vi "Support Get Thermals.vi"(6 "Water Outlet Valve":i32, 8 "error in":errorcluster, 10 "Input Data":T16, 11 "All Data":T1 {"PLC Data"."PLC Data - LDO"."Timing"."Absolute Time" format="%<%H:%M:%S%3u>t"; "PLC Data"."PLC Data - LDO"."Timing"."Display Time" format="%#.20f"; "PLC Data"."PLC Data - LDO"."Timing"."Test Time Ref" format="%#.20f"; "PLC Data"."PLC Data - LDO"."Timing"."Precondition Time Ref" format="%#.20f"; "PLC Data"."PLC Data - LDO"."Timing"."First Call Time Ref" format="%#.20f"; "PLC Data"."PLC Data - FVIR"."Timing"."Absolute Time" format="%<%H:%M:%S%3u>t"; "PLC Data"."PLC Data - FVIR"."Timing"."Display Time" format="%#.20f"; "PLC Data"."PLC Data - FVIR"."Timing"."Test Time Ref" format="%#.20f"; "PLC Data"."PLC Data - FVIR"."Timing"."Precondition Time Ref" format="%#.20f"; "PLC Data"."PLC Data - FVIR"."Timing"."First Call Time Ref" format="%#.20f"}) -> (0 "error out":errorcluster, 3 "All Data Out":T1 {"PLC Data"."PLC Data - LDO"."Timing"."Absolute Time" format="%<%H:%M:%S%3u>t"; "PLC Data"."PLC Data - LDO"."Timing"."Display Time" format="%#.20f"; "PLC Data"."PLC Data - LDO"."Timing"."Test Time Ref" format="%#.20f"; "PLC Data"."PLC Data - LDO"."Timing"."Precondition Time Ref" format="%#.20f"; "PLC Data"."PLC Data - LDO"."Timing"."First Call Time Ref" format="%#.20f"; "PLC Data"."PLC Data - FVIR"."Timing"."Absolute Time" format="%<%H:%M:%S%3u>t"; "PLC Data"."PLC Data - FVIR"."Timing"."Display Time" format="%#.20f"; "PLC Data"."PLC Data - FVIR"."Timing"."Test Time Ref" format="%#.20f"; "PLC Data"."PLC Data - FVIR"."Timing"."Precondition Time Ref" format="%#.20f"; "PLC Data"."PLC Data - FVIR"."Timing"."First Call Time Ref" format="%#.20f"})   [LabVIEW 2023]
uses:
  Modbus/Modbus All Data.ctl
  Modbus/Modbus PLC Data All.ctl
  Modbus/Modbus FVIR Control.ctl
  Modbus/Modbus Timing.ctl
  <vilib>/Utility/miscctls.llb/LVDateTimeRec.ctl
  Modbus/Modbus LDO Control.ctl
  WritingDataFile/Data to Save.ctl
  Terminate Conditions Cluster.ctl
  Drivers/Inficon Transmitter/Type Definitions/Inficon Data.ctl
  Modbus/Modbus Gas Meter Data.ctl
  Drivers/Alicat LabVIEW Drivers 2v1/Sub-VIs/Data Cluster.ctl
  Drivers/Alicat LabVIEW Drivers 2v1/Sub-VIs/Units of Measure.ctl
  Gas_Rate/HEWH ANSI Rate.ctl
  Drivers/Resideo Gas Valve/Type Definitions/Vesta Info.ctl
  Agilent Data.ctl
  Thermal Calculation Cluster.ctl
panel:
  # "Totalizer Timer"
  # "Totalizer Timer"
  # "Natural Gas"
  # "Propane"
  # "Totalizer Timer"
  # "Totalizer Timer"
  # "Natural Gas"
  # "Propane"
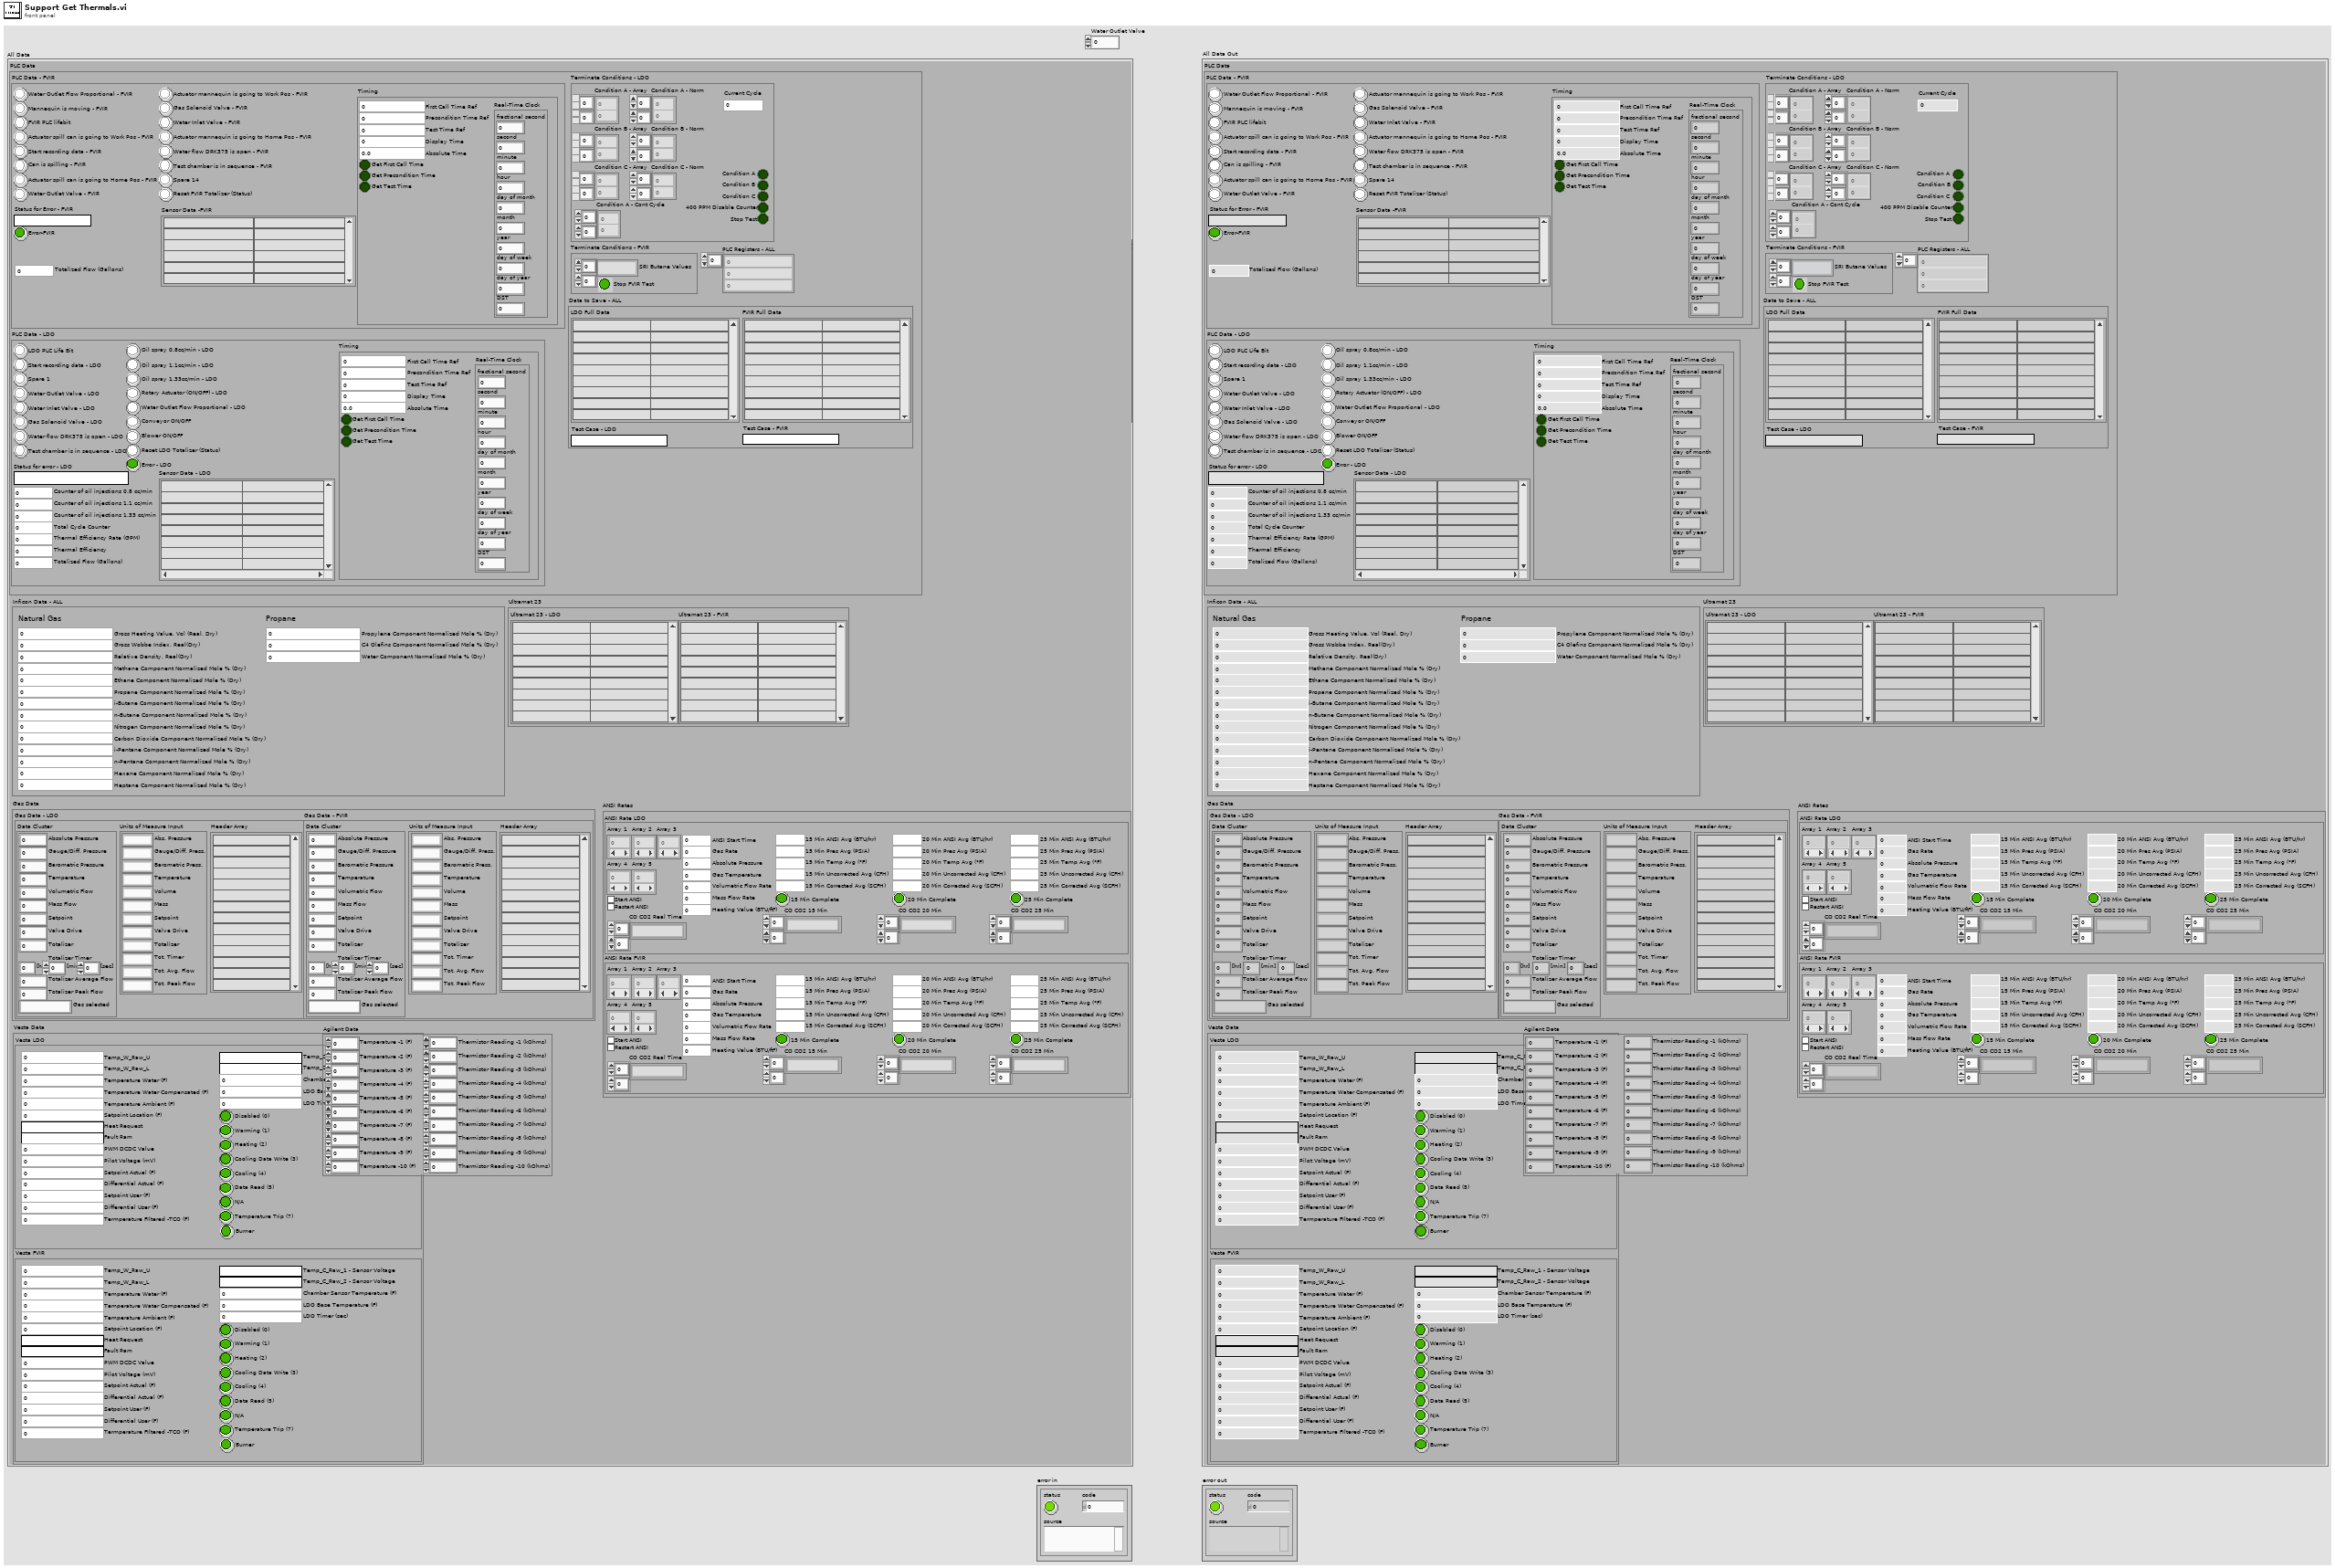
[diagram p1: front panel]
types:
  T1 = typedef "Modbus All Data.ctl" = cluster{"PLC Data":T2, "Inficon Data - ALL":T9, "Gas Data":cluster{"Gas Data - LDO":T10, "Gas Data - FVIR":T10}, "Ultramat 23":cluster{"Ultramat 23 - LDO":string[][], "Ultramat 23 - FVIR":string[][]}, "ANSI Rates":cluster{"ANSI Rate LDO":T13, "ANSI Rate FVIR":T13}, "Vesta Data":cluster{"Vesta LDO":T14, "Vesta FVIR":T14}, "Agilent Data":T15}
  T2 = typedef "Modbus PLC Data All.ctl" = cluster{"PLC Data - FVIR":T3, "PLC Data - LDO":T6, "PLC Registers - ALL":i16[], "Data to Save - ALL":T7, "Terminate Conditions - LDO":T8, "Terminate Conditions - FVIR":cluster{"SRI Butane Values":string[][], "Stop FVIR Test":bool}}
  T3 = typedef "Modbus FVIR Control.ctl" = cluster{"Reset FVIR Totalizer (Status)":bool, "Spare 14":bool, "Actuator mannequin is going to Work Pos - FVIR":bool, "Actuator mannequin is going to Home Pos - FVIR":bool, "Test chamber is in sequence - FVIR ":bool, "Water flow DRK375 is open - FVIR":bool, "Gas Solenoid Valve - FVIR":bool, "Water Inlet Valve - FVIR":bool, "Water Outlet Flow Proportional - FVIR":bool, "Start recording data - FVIR":bool, "Actuator spill can is going to Work Pos - FVIR":bool, "Actuator spill can is going to Home Pos - FVIR":bool, "Water Outlet Valve - FVIR":bool, "Can is spilling - FVIR":bool, "Mannequin is moving - FVIR":bool, "FVIR PLC lifebit":bool, "Status for Error - FVIR":string, "Error-FVIR":bool, "Sensor Data -FVIR":string[][], "Totalized Flow (Gallons)":dbl, "Timing":T4}
  T4 = typedef "Modbus Timing.ctl" = cluster{"First Call Time Ref":dbl, "Precondition Time Ref":dbl, "Test Time Ref":dbl, "Get First Call Time":bool, "Get Precondition Time":bool, "Get Test Time":bool, "Display Time":dbl, "Real-Time Clock":T5, "Absolute Time":dbl}
  T5 = typedef "LVDateTimeRec.ctl" = cluster{"fractional second":dbl, "second":i32, "minute":i32, "hour":i32, "day of month":i32, "month":i32, "year":i32, "day of week":i32, "day of year":i32, "DST":i32}
  T6 = typedef "Modbus LDO Control.ctl" = cluster{"LDO PLC Life Bit":bool, "Start recording data - LDO":bool, "Spare 1":bool, "Water Outlet Valve - LDO":bool, "Water Inlet Valve - LDO":bool, "Gas Solenoid Valve - LDO":bool, "Water flow DRK375 is open - LDO":bool, "Test chamber is in sequence - LDO":bool, "Oil spray 0.8cc/min - LDO":bool, "Oil spray 1.1cc/min - LDO":bool, "Oil spray 1.33cc/min - LDO":bool, "Rotary Actuator (ON/OFF) - LDO":bool, "Water Outlet Flow Proportional - LDO":bool, "Conveyor ON/OFF":bool, "Blower ON/OFF":bool, "Reset LDO Totalizer (Status)":bool, "Status for error - LDO":string, "Error - LDO":bool, "Sensor Data - LDO":string[][], "Thermal Efficiency Rate (GPM)":dbl, "Thermal Efficiency":dbl, "Totalized Flow (Gallons)":dbl, "Counter of oil injections 1.33 cc/min":u16, "Total Cycle Counter":u16, "Counter of oil injections 1.1 cc/min":u16, "Counter of oil injections 0.8 cc/min":u16, "Timing":T4}
  T7 = typedef "Data to Save.ctl" = cluster{"LDO Full Data":string[][], "FVIR Full Data":string[][], "Test Case - FVIR":string, "Test Case - LDO":string}
  T8 = typedef "Terminate Conditions Cluster.ctl" = cluster{"Condition B - Array":dbl[][], "Current Cycle":u16, "Condition C - Array":dbl[][], "Condition A - Array":dbl[][], "400 PPM Disable Counter":bool, "Condition A - Norm":dbl[][], "Condition B - Norm":dbl[][], "Condition C - Norm":dbl[][], "Condition A":bool, "Condition B":bool, "Condition C":bool, "Condition A - Cont Cycle":dbl[][], "Stop Test":bool}
  T9 = typedef "Inficon Data.ctl" = cluster{"Gross Heating Value, Vol (Real, Dry)":dbl, "Nitrogen Component Normalized Mole % (Dry)":dbl, "Methane Component Normalized Mole % (Dry)":dbl, "Carbon Dioxide Component Normalized Mole % (Dry)":dbl, "Ethane Component Normalized Mole % (Dry)":dbl, "Propane Component Normalized Mole % (Dry)":dbl, "i-Pentane Component Normalized Mole % (Dry)":dbl, "i-Butane Component Normalized Mole % (Dry)":dbl, "n-Butane Component Normalized Mole % (Dry)":dbl, "n-Pentane Component Normalized Mole % (Dry)":dbl, "Hexane Component Normalized Mole % (Dry)":dbl, "Heptane Component Normalized Mole % (Dry)":dbl, "Gross Wobbe Index, Real(Dry)":dbl, "Relative Density, Real(Dry)":dbl, "Propylene Component Normalized Mole % (Dry)":dbl, "C4 Olefins Component Normalized Mole % (Dry)":dbl, "Water Component Normalized Mole % (Dry)":dbl}
  T10 = typedef "Modbus Gas Meter Data.ctl" = cluster{"Data Cluster":T11, "Units of Measure Input":T12, "Header Array":string[]}
  T11 = typedef "Data Cluster.ctl" = cluster{"Absolute Pressure":dbl, "Gauge/Diff. Pressure":dbl, "Barometric Pressure":dbl, "Temperature":dbl, "Volumetric Flow":dbl, "Mass Flow":dbl, "Setpoint":dbl, "Valve Drive":dbl, "Totalizer":dbl, "[hr]":dbl, "[min]":dbl, "[sec]":dbl, "Totalizer Average Flow":dbl, "Totalizer Peak Flow":dbl, "Gas selected":string}
  T12 = typedef "Units of Measure.ctl" = cluster{"Abs. Pressure":string, "Gauge/Diff. Press.":string, "Barometric Press.":string, "Temperature":string, "Volume":string, "Mass":string, "Setpoint":string, "Valve Drive":string, "Totalizer":string, "Tot. Timer":string, "Tot. Avg. Flow":string, "Tot. Peak Flow":string}
  T13 = typedef "HEWH ANSI Rate.ctl" = cluster{"Array 1":dbl[], "Array 3":dbl[], "Array 2":dbl[], "Start ANSI":bool, "ANSI Start Time":dbl, "Restart ANSI":bool, "15 Min ANSI Avg (BTU/hr)":dbl, "20 Min ANSI Avg (BTU/hr)":dbl, "25 Min ANSI Avg (BTU/hr)":dbl, "Absolute Pressure":dbl, "Gas Temperature":dbl, "Volumetric Flow Rate":dbl, "Mass Flow Rate":dbl, "Array 4":dbl[], "Array 5":dbl[], "Gas Rate":dbl, "15 Min Pres Avg (PSIA)":dbl, "20 Min Pres Avg (PSIA)":dbl, "25 Min Pres Avg (PSIA)":dbl, "15 Min Temp Avg (°F) ":dbl, "20 Min Temp Avg (°F)":dbl, "25 Min Temp Avg (°F)":dbl, "15 Min Uncorrected Avg (CFH)":dbl, "20 Min Uncorrected Avg (CFH)":dbl, "25 Min Uncorrected Avg (CFH)":dbl, "15 Min Corrected Avg (SCFH)":dbl, "20 Min Corrected Avg (SCFH)":dbl, "25 Min Corrected Avg (SCFH)":dbl, "15 Min Complete":bool, "20 Min Complete":bool, "25 Min Complete":bool, "Heating Value (BTU/ft³)":dbl, "CO CO2 15 Min":string[][], "CO CO2 20 Min":string[][], "CO CO2 25 Min":string[][], "CO CO2 Real Time":string[][]}
  T14 = typedef "Vesta Info.ctl" = cluster{"Temp_W_Raw_U":u16, "Temp_W_Raw_L":u16, "Temperature Water (F)":dbl, "Temperature Water Compensated (F)":dbl, "Temperature Ambient (F)":dbl, "Setpoint Location (F)":dbl, "Heat Request":string, "Fault Ram":string, "PWM DCDC Value":u16, "Pilot Voltage (mV)":dbl, "Setpoint Actual (F)":dbl, "Differential Actual (F)":dbl, "Setpoint User (F)":dbl, "Differential User (F)":dbl, "Termperature FIltered -TCO (F)":dbl, "Temp_C_Raw_1 - Sensor Voltage":string, "Temp_C_Raw_2 - Sensor Voltage":string, "Chamber Sensor Temperature (F)":dbl, "LDO Base Temperature (F)":dbl, "LDO Timer (sec)":i16, "Disabled (0)":bool, "Warming (1)":bool, "Heating (2)":bool, "Cooling Data Write (3)":bool, "Cooling (4)":bool, "Data Read (5)":bool, "N/A":bool, "Temperature Trip (7)":bool, "Burner":bool}
  T15 = typedef "Agilent Data.ctl" = cluster{"Temperature -1 (F)":dbl, "Thermistor Reading -1 (kOhms)":dbl, "Thermistor Reading -2 (kOhms)":dbl, "Temperature -2 (F)":dbl, "Thermistor Reading -3 (kOhms)":dbl, "Temperature -3 (F)":dbl, "Thermistor Reading -4 (kOhms)":dbl, "Temperature -4 (F)":dbl, "Thermistor Reading -5 (kOhms)":dbl, "Temperature -5 (F)":dbl, "Thermistor Reading -6 (kOhms)":dbl, "Temperature -6 (F)":dbl, "Thermistor Reading -7 (kOhms)":dbl, "Temperature -7 (F)":dbl, "Thermistor Reading -8 (kOhms)":dbl, "Temperature -8 (F)":dbl, "Thermistor Reading -9 (kOhms)":dbl, "Temperature -9 (F)":dbl, "Thermistor Reading -10 (kOhms)":dbl, "Temperature -10 (F)":dbl}
  T16 = typedef "Thermal Calculation Cluster.ctl" = cluster{"Gross Heating Value, Vol (Real, Dry)":dbl, "RTD Out (Deg F)":dbl, "RTD In (Deg F)":dbl, "Gallons (Gal)":dbl, "Gas Mass Flow":dbl, "Gas Totalizer":dbl, "Use Constant Thermal Efficiency":bool, "Constant Thermal Eff":dbl}
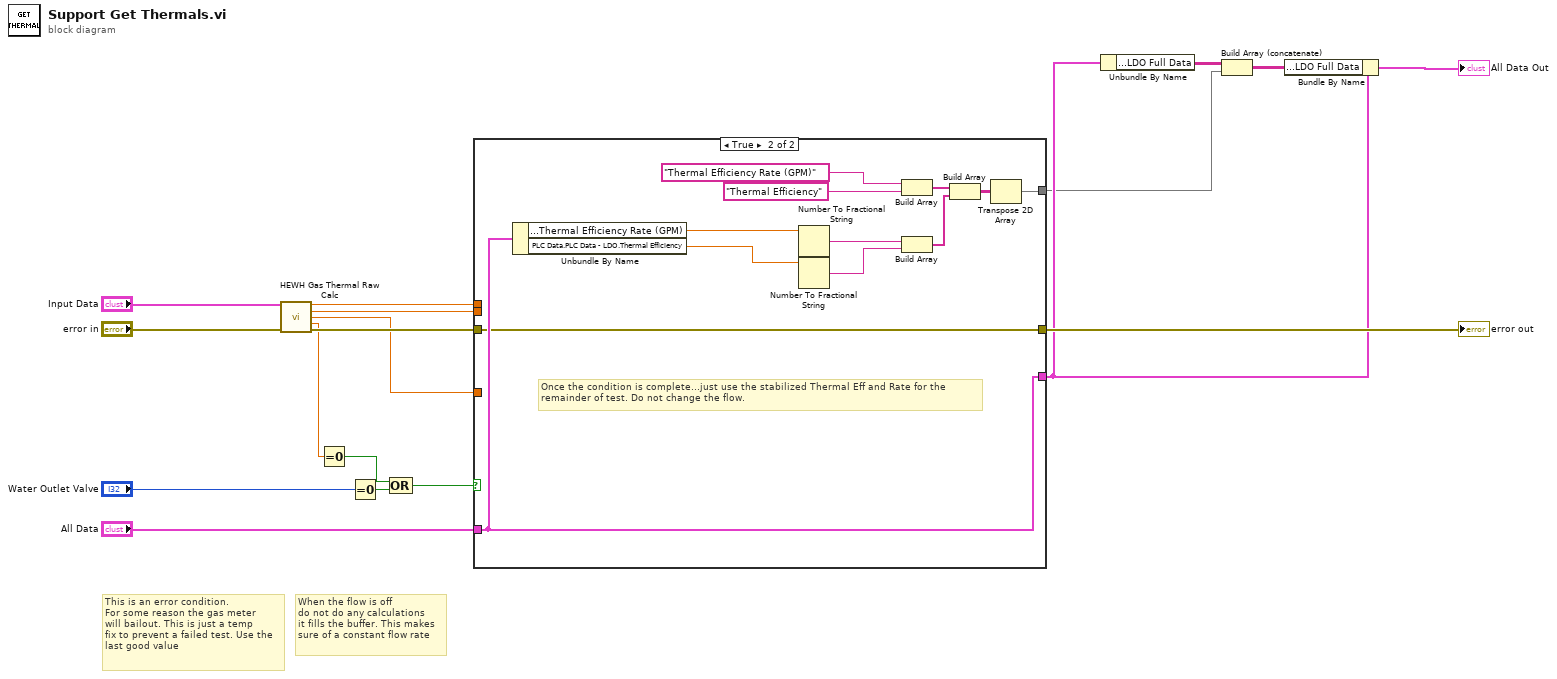
[diagram p0: block diagram]
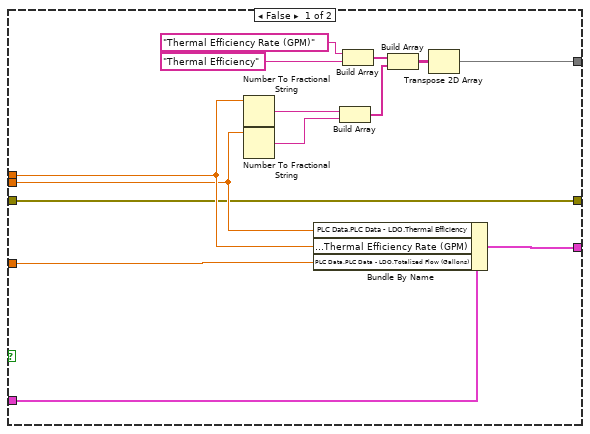
[diagram p2: hidden frame]
diagram:
  # "When the flow is off\ndo not do any calculations\nit fills the buffer. This makes\nsure of a constant flow rate"
  # "This is an error condition.\nFor some reason the gas meter \nwill bailout. This is just a temp\nfix to prevent a failed test. Use the\nlast good value"
  n1 = call "HEWH Gas Thermal Raw Calc.vi"("Input Data"="Input Data", "error in (no error)"="error in") -> ("Rate"=w9:dbl, "Eff"=w10:dbl, "Gallons (Gal)"=w6:dbl, "Gas Mass Flow"=w7:dbl, "error out"=w11:errorcluster)  [unwired: 9 in]
  n2 = Equal To 0?(x=w7) -> (x = 0?=w14:bool)
  n3 = Equal To 0?(x="Water Outlet Valve") -> (x = 0?=w15:bool)
  n4 = Compound Arithmetic op=OR(w14, w15) -> (w16:bool)
  n5 = case shown="True" w16 {
    tunnel: [w25 w34] -> w1
    tunnel: w9 -> [w24 _]
    tunnel: [w23 w44] -> w3
    tunnel: w10 -> [w22 _]
    tunnel: w6 -> [w21 _]
    tunnel: "All Data" -> [w20 w44]
    tunnel: w11 -> [w19 w33]
    tunnel: [w19 w33] -> w12
    frame False {
      n6 = Number To Fractional String(number=w24) -> (F-format string=w32:string)  [unwired: 3 in]
      n7 = Number To Fractional String(number=w22) -> (F-format string=w31:string)  [unwired: 3 in]
      n8 = Bundle By Name(cluster=w20, "PLC Data.PLC Data - LDO.Thermal Efficiency"=w22, "PLC Data.PLC Data - LDO.Thermal Efficiency Rate (GPM)"=w24, "PLC Data.PLC Data - LDO.Totalized Flow (Gallons)"=w21) -> (w23:T1)
      n9 = Build Array(w32, w31) -> (w28:string[])
      n10 = Build Array("Thermal Efficiency Rate (GPM)", "Thermal Efficiency") -> (w27:string[])
      n11 = Build Array(w27, w28) -> (w26:string[][])
      n12 = Transpose 2D Array(2D array=w26) -> (transposed array=w25:string[][])
    }
    frame True {
      # "Once the condition is complete...just use the stabilized Thermal Eff and Rate for the \nremainder of test. Do not change the flow."
      n13 = Unbundle By Name(w44) -> ("PLC Data.PLC Data - LDO.Thermal Efficiency Rate (GPM)"=w36:dbl, "PLC Data.PLC Data - LDO.Thermal Efficiency"=w35:dbl)
      n14 = Number To Fractional String(number=w36) -> (F-format string=w43:string)  [unwired: 3 in]
      n15 = Number To Fractional String(number=w35) -> (F-format string=w42:string)  [unwired: 3 in]
      n16 = Build Array("Thermal Efficiency Rate (GPM)", "Thermal Efficiency") -> (w40:string[])
      n17 = Build Array(w43, w42) -> (w41:string[])
      n18 = Build Array(w40, w41) -> (w39:string[][])
      n19 = Transpose 2D Array(2D array=w39) -> (transposed array=w34:string[][])
    }
  }
  "error out" <- w12
  n20 = Unbundle By Name(w3) -> ("PLC Data.Data to Save - ALL.LDO Full Data"=w4:string[][])
  n21 = Build Array (concatenate)(w4, w1) -> (w2:string[][])
  n22 = Bundle By Name(cluster=w3, "PLC Data.Data to Save - ALL.LDO Full Data"=w2) -> (→"All Data Out":T1)
